vi "Initialise.vi"(6 "ProjectPath":path, 8 "error in (no error)":errorcluster, 11 "Interface Name":string) -> (0 "error out":errorcluster, 3 "CreateInterface out":refnum<class "CreateInterface.lvclass">)   [LabVIEW 2020, in "Mermaid.lvlib" / "CreateInterface.lvclass"]
uses:
  CreateInterface.lvclass
  CreateInterface.lvclass/CreateInterface.ctl
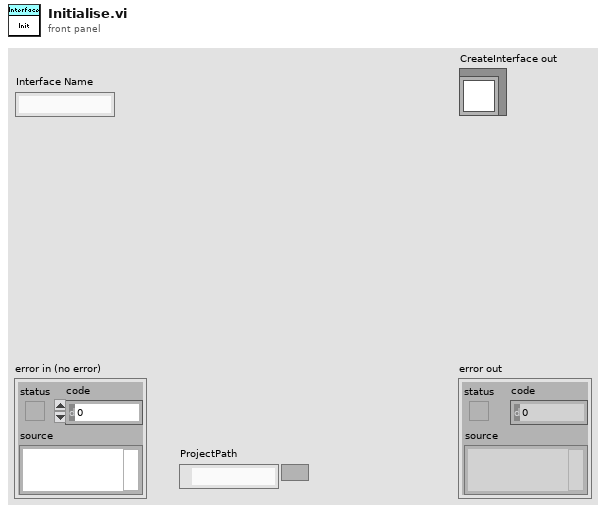
[diagram p1: front panel]
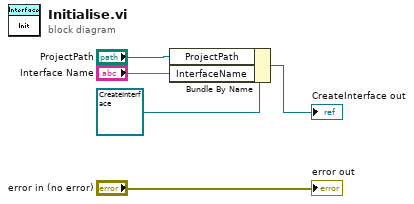
[diagram p0: block diagram]
diagram:
  n1 = Bundle By Name(cluster=refnum<class "CreateInterface.lvclass"> refnum ("CreateInterface out"), "ProjectPath"="ProjectPath", "InterfaceName"="Interface Name") -> (→"CreateInterface out":refnum<class "CreateInterface.lvclass">)
  "error out" <- "error in (no error)"
